vi "Registration Complete.vi"(8 "error in (no error)":errorcluster, 11 "EventHandler":refnum<class "IEventHandler.lvclass">) -> (0 "error out":errorcluster, 3 "EventHandler":refnum<class "IEventHandler.lvclass">)   [LabVIEW 2015, in "ActorEvents.lvlib" / "IEventHandler.lvclass"]
uses:
  IEventHandler.lvclass
  IEventHandler.lvclass/IEventHandler.ctl
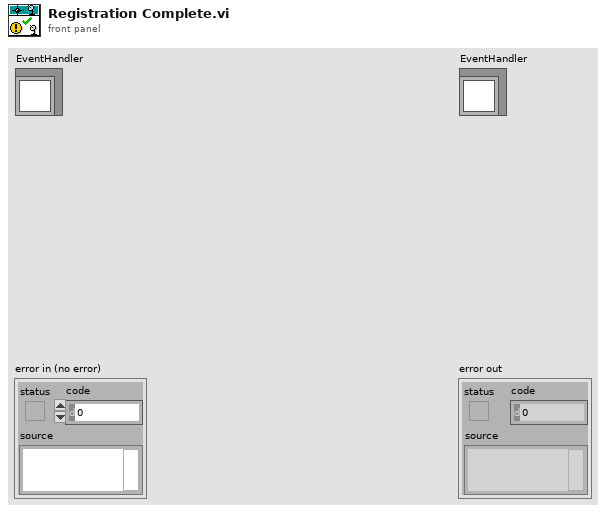
[diagram p1: front panel]
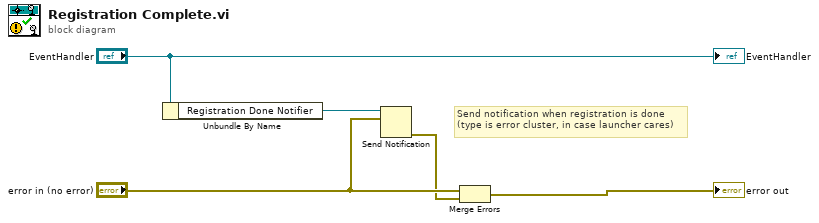
[diagram p0: block diagram]
diagram:
  # "Send notification when registration is done\n(type is error cluster, in case launcher cares)"
  n1 = Unbundle By Name("EventHandler") -> ("Registration Done Notifier"=w4:refnum<notifier>)
  n2 = Send Notification(notification="error in (no error)", notifier=w4) -> (error out=w1:errorcluster)  [unwired: 1 in, 1 out]
  n3 = Merge Errors("error in (no error)", w1) -> (→"error out":errorcluster)
  "EventHandler" <- "EventHandler"
